vi "_API_BINANCE_DELETE_USDT_FUTURES_DeleteCurrentAllOpenOrders.vi"(0 "BinanceAPI in":refnum<class "BinanceAPI_.lvclass">, 5 "CurrentAllOpenOrders":cluster{"symbol (eg. BTCUSDT)":string}, 11 "error in (no error)":errorcluster) -> (4 "BinanceAPI out":refnum<class "BinanceAPI_.lvclass">, 14 "Body":string, 15 "error out":errorcluster)   [LabVIEW 2022 SP3, in "BinanceAPI_.lvclass"]
doc: "https://binance-docs.github.io/apidocs/futures/en/#cancel-all-open-orders-trade"
uses:
  BinanceAPI_.lvclass
  BinanceAPI_.lvclass/BinanceAPI_.ctl
panel:
  out "Header":string
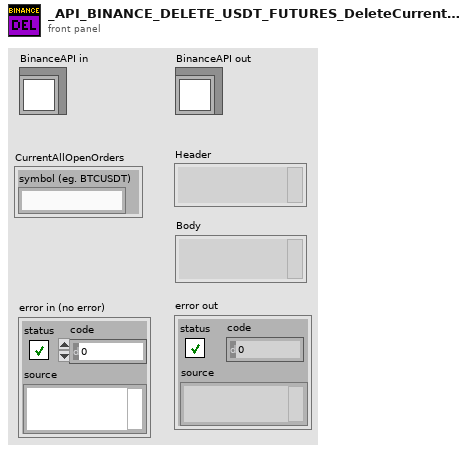
[diagram p1: front panel]
types:
  T1 = enum16{"SPOT", "USDT_FUTURES", "COIN_FUTURES", "VANILLA"}
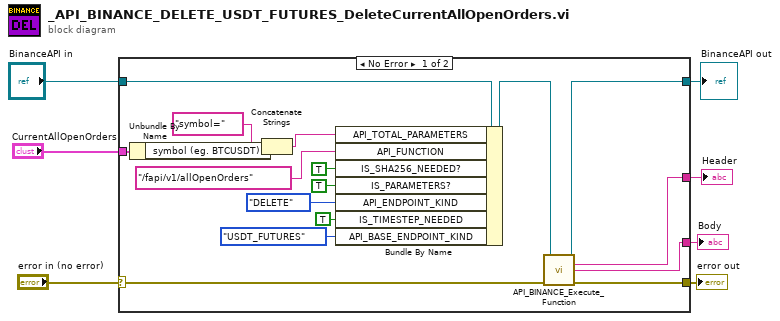
[diagram p0: block diagram]
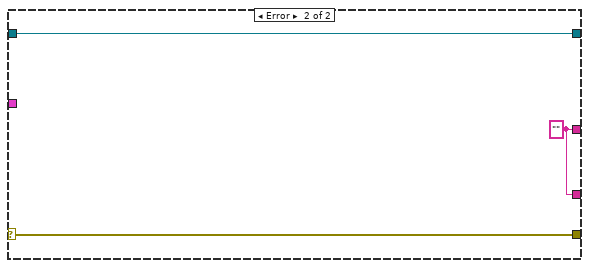
[diagram p2: hidden frame]
diagram:
  n1 = case shown="No Error" "error in (no error)" {
    selector: "error in (no error)" -> [w13 w27]
    tunnel: [w12 w27] -> w5
    tunnel: [w14 w26] -> w1
    tunnel: "BinanceAPI in" -> [w24 w26]
    tunnel: "CurrentAllOpenOrders" -> [w17 _]
    tunnel: [w9 w25] -> w4
    tunnel: [w8 w25] -> w3
    frame No Error {
      n2 = Unbundle By Name(w17) -> ("symbol (eg. BTCUSDT)"=w16:string)
      n3 = Concatenate Strings("symbol=", w16) -> (w18:string)
      n4 = Bundle By Name(cluster=w24, "API_TOTAL_PARAMETERS"=w18, "API_FUNCTION"="/fapi/v1/allOpenOrders", "IS_SHA256_NEEDED?"=TRUE, "IS_PARAMETERS?"=TRUE, "API_ENDPOINT_KIND"=enum16{"POST", "DELETE", "GET", "PUT"}."DELETE", "IS_TIMESTEP_NEEDED"=TRUE, "API_BASE_ENDPOINT_KIND"=T1."USDT_FUTURES") -> (w15:refnum<class "BinanceAPI_.lvclass">)
      n5 = call "API_BINANCE_Execute_Function.vi"("BinanceAPI in"=w15, "error in (no error)"=w13) -> ("BinanceAPI out"=w14:refnum<class "BinanceAPI_.lvclass">, "Header"=w9:string, "Body"=w8:string, "error out"=w12:errorcluster)  [unwired: 9 in, 1 out]
    }
    frame Error {
      w25 = "" ("Header")
    }
  }
  "error out" <- w5
  "Body" <- w3
  "Header" <- w4
  "BinanceAPI out" <- w1
